vi "Scan SN.vi"() -> (1 "Continue":bool, 2 "SN_Array":string[](array[string]), 3 "ActiveUUT":bool[](array[boolean]))   [LabVIEW 2023]
panel:
  in  "Start":bool caption="Play"
  in  "Cancel Button":bool
  in  "UUT 4":string
  in  "UUT 3":string
  in  "UUT 2":string
  in  "UUT 1":string
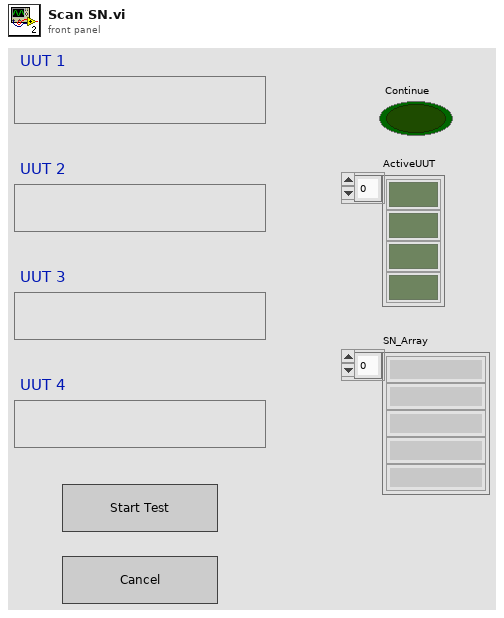
[diagram p1: front panel]
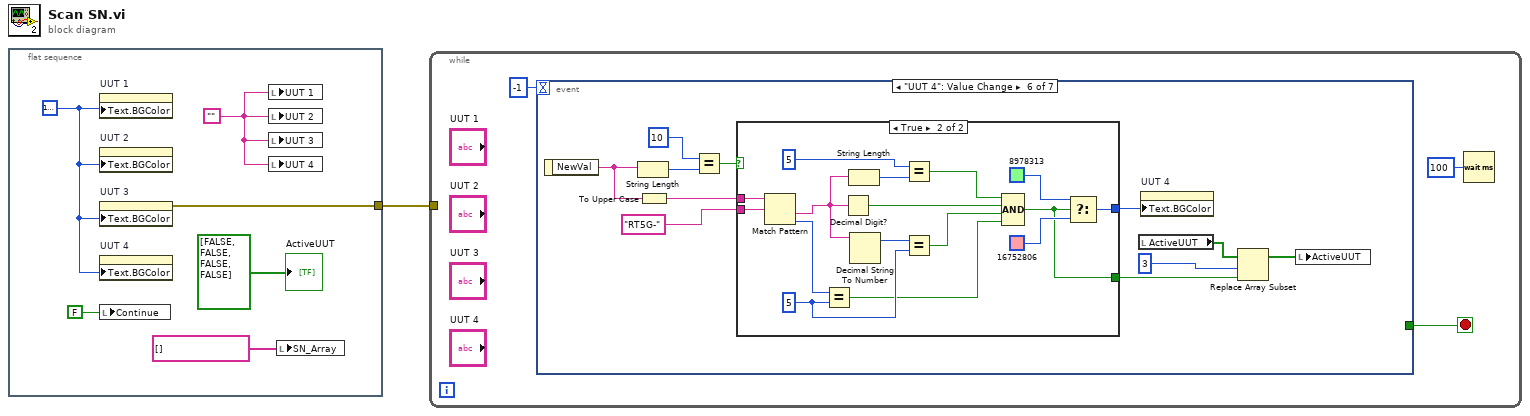
[diagram p0: block diagram]
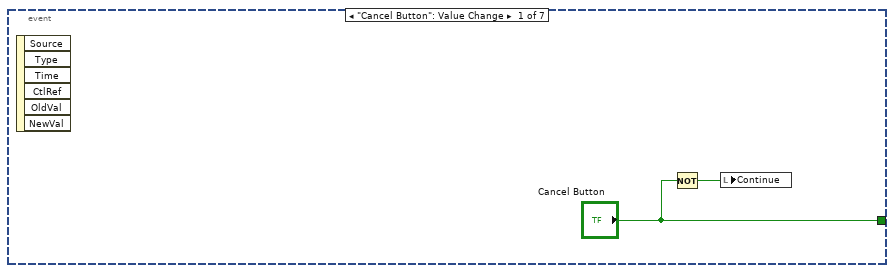
[diagram p2: hidden frame]
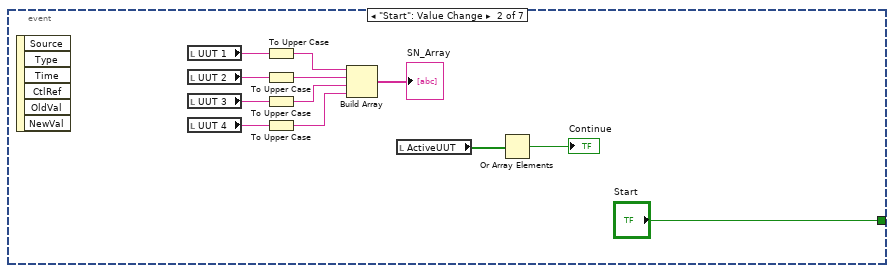
[diagram p3: hidden frame]
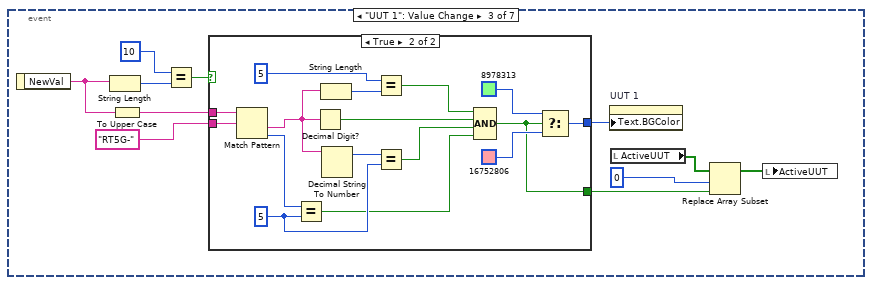
[diagram p4: hidden frame]
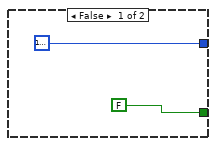
[diagram p5: hidden frame]
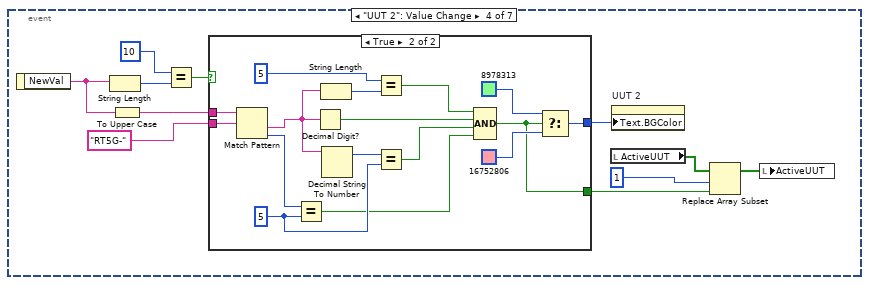
[diagram p6: hidden frame]
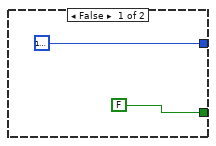
[diagram p7: hidden frame]
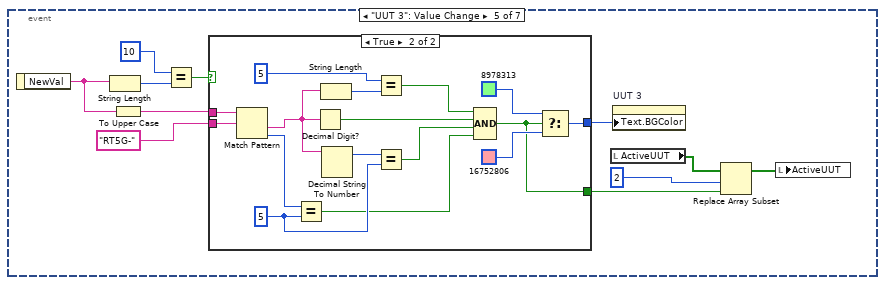
[diagram p8: hidden frame]
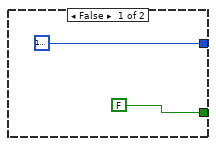
[diagram p9: hidden frame]
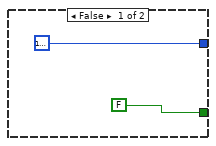
[diagram p10: hidden frame]
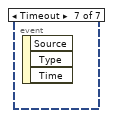
[diagram p11: hidden frame]
diagram:
  n1 = flat-sequence {
    tunnel: [w5] -> w1
    frame #0 {
      w6 = ""
      w7 = u32 16777225 ("Text.Text Colors:BG Color")
      n2 = property on="UUT 1" class="Str"("Text.BGColor"=w7) -> ()  [unwired: 2 in, 2 out]
      n3 = property on="UUT 2" class="Str"("Text.BGColor"=w7) -> ()  [unwired: 2 in, 2 out]
      n4 = property on="UUT 3" class="Str"("Text.BGColor"=w7) -> (error out=w5:errorcluster)  [unwired: 2 in, 1 out]
      n5 = property on="UUT 4" class="Str"("Text.BGColor"=w7) -> ()  [unwired: 2 in, 2 out]
      n6 = local write "Continue"(FALSE ("Continue")) -> ()
      n7 = local write "UUT 1"(w6) -> ()
      n8 = local write "UUT 2"(w6) -> ()
      n9 = local write "UUT 3"(w6) -> ()
      n10 = local write "UUT 4"(w6) -> ()
      n11 = local write "SN_Array"(string[] [] ("SN_Array")) -> ()
      "ActiveUUT" <- bool[] [FALSE, FALSE, FALSE, FALSE]
    }
  }
  n12 = while {
    tunnel: w1 -> [_]
    stop <- w9 stop-if-true
    n13 = event shown="[5] \"UUT 4\": Value Change" {
      selector: _ -> [_ _ _ _ _ _ _]
      dyn-events: _ -> [_ _ _ _ _ _ _]
      timeout: -1 -> [_ _ _ _ _ _ _]
      tunnel: ["Cancel Button" "Start" _ _ _ _ _] -> w9
      event "Cancel Button": Value Change {
        n14 = event-data() -> ()  [unwired: 1 in, 6 out]
        n15 = Not(x="Cancel Button") -> (.not. x?=w11:bool)
        n16 = local write "Continue"(w11) -> ()
      }
      event "Start": Value Change {
        n17 = event-data() -> ()  [unwired: 1 in, 6 out]
        n18 = local read "UUT 1"() -> (w16:string)
        n19 = local read "UUT 2"() -> (w17:string)
        n20 = local read "UUT 3"() -> (w18:string)
        n21 = local read "UUT 4"() -> (w19:string)
        n22 = To Upper Case(1:w16) -> (0:w20:string)
        n23 = To Upper Case(1:w17) -> (0:w21:string)
        n24 = To Upper Case(1:w18) -> (0:w22:string)
        n25 = To Upper Case(1:w19) -> (0:w23:string)
        n26 = Build Array(w20, w21, w22, w23) -> (→"SN_Array":string[])
        n27 = local read "ActiveUUT"() -> (w14:bool[])
        n28 = Or Array Elements(Boolean array=w14) -> (logical OR=→"Continue":bool)
      }
      event "UUT 1": Value Change {
        n29 = event-data() -> ("NewVal"=w27:string)  [unwired: 1 in]
        n30 = String Length(string=w27) -> (length=w35:i32)
        n31 = To Upper Case(1:w27) -> (0:w26:string)
        n32 = Equal?(x=10, y=w35) -> (x = y?=w33:bool)
        n33 = case shown="True" w33 {
          tunnel: w26 -> [_ w52]
          tunnel: "RT5G-" -> [_ w51]
          tunnel: [u32 16777225 ("Text.Text Colors:BG Color") w44] -> w31
          tunnel: [FALSE w38] -> w29
          frame False {
          }
          frame True {
            w42 = 5 ("y")
            n34 = Match Pattern(string=w52, regular expression=w51) -> (after substring=w39:string, offset past match=w53:i32)  [unwired: 1 in, 2 out]
            n35 = Equal?(x=w53, y=w42) -> (x = y?=w41:bool)
            n36 = Decimal Digit?(1:w39) -> (0:w48:bool)
            n37 = String Length(string=w39) -> (length=w50:i32)
            n38 = Decimal String To Number(string=w39) -> (offset past number=w43:i32)  [unwired: 2 in, 1 out]
            n39 = Equal?(x=5 ("y"), y=w50) -> (x = y?=w47:bool)
            n40 = Equal?(x=w43, y=w42) -> (x = y?=w40:bool)
            n41 = Compound Arithmetic op=AND(w47, w48, w40, w41) -> (w38:bool)
            n42 = Select(t=u32 8978313 ("Text.Text Colors:BG Color"), s=w38, f=u32 16752806 ("Text.Text Colors:BG Color")) -> (s? t:f=w44:u32)
          }
        }
        n43 = property on="UUT 1" class="Str"("Text.BGColor"=w31) -> ()  [unwired: 2 in, 2 out]
        n44 = local read "ActiveUUT"() -> (w30:bool[])
        n45 = Replace Array Subset(array=w30, new element=w29, index=0) -> (w25:bool[])
        n46 = local write "ActiveUUT"(w25) -> ()
      }
      event "UUT 2": Value Change {
        n47 = event-data() -> ("NewVal"=w56:string)  [unwired: 1 in]
        n48 = String Length(string=w56) -> (length=w64:i32)
        n49 = To Upper Case(1:w56) -> (0:w55:string)
        n50 = Equal?(x=10, y=w64) -> (x = y?=w62:bool)
        n51 = case shown="True" w62 {
          tunnel: w55 -> [_ w81]
          tunnel: "RT5G-" -> [_ w80]
          tunnel: [u32 16777225 ("Text.Text Colors:BG Color") w73] -> w57
          tunnel: [FALSE w67] -> w59
          frame False {
          }
          frame True {
            w71 = 5 ("y")
            n52 = Match Pattern(string=w81, regular expression=w80) -> (after substring=w68:string, offset past match=w82:i32)  [unwired: 1 in, 2 out]
            n53 = Equal?(x=w82, y=w71) -> (x = y?=w70:bool)
            n54 = Decimal Digit?(1:w68) -> (0:w77:bool)
            n55 = String Length(string=w68) -> (length=w79:i32)
            n56 = Decimal String To Number(string=w68) -> (offset past number=w72:i32)  [unwired: 2 in, 1 out]
            n57 = Equal?(x=5 ("y"), y=w79) -> (x = y?=w76:bool)
            n58 = Equal?(x=w72, y=w71) -> (x = y?=w69:bool)
            n59 = Compound Arithmetic op=AND(w76, w77, w69, w70) -> (w67:bool)
            n60 = Select(t=u32 8978313 ("Text.Text Colors:BG Color"), s=w67, f=u32 16752806 ("Text.Text Colors:BG Color")) -> (s? t:f=w73:u32)
          }
        }
        n61 = local read "ActiveUUT"() -> (w60:bool[])
        n62 = property on="UUT 2" class="Str"("Text.BGColor"=w57) -> ()  [unwired: 2 in, 2 out]
        n63 = Replace Array Subset(array=w60, new element=w59, index=1) -> (w54:bool[])
        n64 = local write "ActiveUUT"(w54) -> ()
      }
      event "UUT 3": Value Change {
        n65 = event-data() -> ("NewVal"=w85:string)  [unwired: 1 in]
        n66 = String Length(string=w85) -> (length=w93:i32)
        n67 = To Upper Case(1:w85) -> (0:w84:string)
        n68 = Equal?(x=10, y=w93) -> (x = y?=w91:bool)
        n69 = case shown="True" w91 {
          tunnel: w84 -> [_ w110]
          tunnel: "RT5G-" -> [_ w109]
          tunnel: [u32 16777225 ("Text.Text Colors:BG Color") w102] -> w89
          tunnel: [FALSE w96] -> w86
          frame False {
          }
          frame True {
            w100 = 5 ("y")
            n70 = Match Pattern(string=w110, regular expression=w109) -> (after substring=w97:string, offset past match=w111:i32)  [unwired: 1 in, 2 out]
            n71 = Equal?(x=w111, y=w100) -> (x = y?=w99:bool)
            n72 = Decimal Digit?(1:w97) -> (0:w106:bool)
            n73 = String Length(string=w97) -> (length=w108:i32)
            n74 = Decimal String To Number(string=w97) -> (offset past number=w101:i32)  [unwired: 2 in, 1 out]
            n75 = Equal?(x=5 ("y"), y=w108) -> (x = y?=w105:bool)
            n76 = Equal?(x=w101, y=w100) -> (x = y?=w98:bool)
            n77 = Compound Arithmetic op=AND(w105, w106, w98, w99) -> (w96:bool)
            n78 = Select(t=u32 8978313 ("Text.Text Colors:BG Color"), s=w96, f=u32 16752806 ("Text.Text Colors:BG Color")) -> (s? t:f=w102:u32)
          }
        }
        n79 = local read "ActiveUUT"() -> (w88:bool[])
        n80 = property on="UUT 3" class="Str"("Text.BGColor"=w89) -> ()  [unwired: 2 in, 2 out]
        n81 = Replace Array Subset(array=w88, new element=w86, index=2) -> (w83:bool[])
        n82 = local write "ActiveUUT"(w83) -> ()
      }
      event "UUT 4": Value Change {
        n83 = event-data() -> ("NewVal"=w114:string)  [unwired: 1 in]
        n84 = String Length(string=w114) -> (length=w122:i32)
        n85 = To Upper Case(1:w114) -> (0:w113:string)
        n86 = Equal?(x=10, y=w122) -> (x = y?=w120:bool)
        n87 = case shown="True" w120 {
          tunnel: w113 -> [_ w139]
          tunnel: "RT5G-" -> [_ w138]
          tunnel: [u32 16777225 ("Text.Text Colors:BG Color") w131] -> w115
          tunnel: [FALSE w125] -> w117
          frame False {
          }
          frame True {
            w129 = 5 ("y")
            n88 = Match Pattern(string=w139, regular expression=w138) -> (after substring=w126:string, offset past match=w140:i32)  [unwired: 1 in, 2 out]
            n89 = Equal?(x=w140, y=w129) -> (x = y?=w128:bool)
            n90 = Decimal Digit?(1:w126) -> (0:w135:bool)
            n91 = String Length(string=w126) -> (length=w137:i32)
            n92 = Decimal String To Number(string=w126) -> (offset past number=w130:i32)  [unwired: 2 in, 1 out]
            n93 = Equal?(x=5 ("y"), y=w137) -> (x = y?=w134:bool)
            n94 = Equal?(x=w130, y=w129) -> (x = y?=w127:bool)
            n95 = Compound Arithmetic op=AND(w134, w135, w127, w128) -> (w125:bool)
            n96 = Select(t=u32 8978313 ("Text.Text Colors:BG Color"), s=w125, f=u32 16752806 ("Text.Text Colors:BG Color")) -> (s? t:f=w131:u32)
          }
        }
        n97 = local read "ActiveUUT"() -> (w118:bool[])
        n98 = property on="UUT 4" class="Str"("Text.BGColor"=w115) -> ()  [unwired: 2 in, 2 out]
        n99 = Replace Array Subset(array=w118, new element=w117, index=3) -> (w112:bool[])
        n100 = local write "ActiveUUT"(w112) -> ()
      }
      event Timeout {
        n101 = event-data() -> ()  [unwired: 1 in, 3 out]
      }
    }
    n102 = Wait (ms)(milliseconds to wait=u32 100) -> ()  [unwired: 1 out]
  }
